vi "_CSMObj-Obtain Worker Agent.vi"(7 "Allowed Messages (Empty For All)":string[](array[string]), 8 "error in (no error)":errorcluster, 11 "Requested Name":string) -> (0 "error out":errorcluster, 3 "CSMQ Out":T1)   [LabVIEW 2017, in "Communicable State Machine.lvlib"]
uses:
  Communicable State Machine.lvlib
  _CSMObj.ctl
  _CSMObj-Info.ctl
  Typedef/_CSM_MODE.ctl
  _CSMObj-Refs.ctl
  _CSMObj-Data.ctl
  Priority Queue/Priority Queue.ctl
  Typedef/_Cross CSM State Data.ctl
  Typedef/_CSM_MSG_TYPE.ctl
  Typedef/_Cross CSM State Response.ctl
  Typedef/_CSM_Response Source Message.ctl
  Priority Queue/def-Data(LowPRI-Q).ctl
  _CSMObj-ModeData.ctl
  Typedef/_CSM Status Change Event Data.ctl
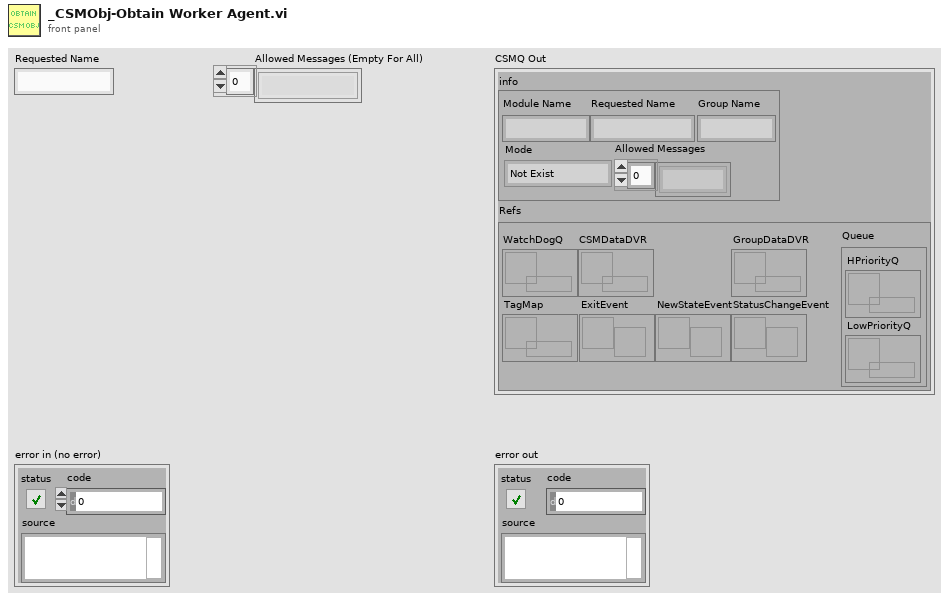
[diagram p1: front panel]
types:
  T1 = typedef "Communicable State Machine.lvlib/_CSMObj.ctl" = cluster{"info":T2, "Refs":T4}
  T2 = typedef "Communicable State Machine.lvlib/_CSMObj-Info.ctl" = cluster{"Module Name":string, "Requested Name":string, "Group Name":string, "Mode":T3, "Allowed Messages":string[]}
  T3 = typedef "Communicable State Machine.lvlib/_CSM_MODE.ctl" = enum16{"Not Exist", "Stand Alone", "CSM", "Worker", "Worker Agent", "Chain Node", "Chain"}
  T4 = typedef "Communicable State Machine.lvlib/_CSMObj-Refs.ctl" = cluster{"WatchDogQ":refnum<queue>, "CSMDataDVR":refnum<data-value>, "Queue":T5, "GroupDataDVR":refnum<data-value>, "TagMap":refnum<data-value>, "ExitEvent":refnum<user-event>, "NewStateEvent":refnum<user-event>, "StatusChangeEvent":refnum<user-event>}
  T5 = typedef "Communicable State Machine.lvlib/Priority Queue.ctl" = cluster{"HPriorityQ":refnum<queue>, "LowPriorityQ":refnum<queue>}
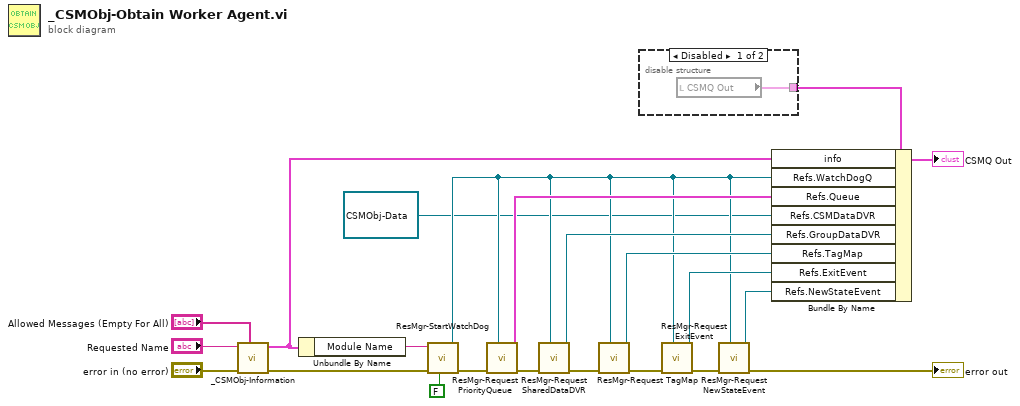
[diagram p0: block diagram]
diagram:
  n1 = call "_CSMObj-Information.vi"("Allowed Messages (Empty For All)"="Allowed Messages (Empty For All)", "Error In"="error in (no error)", "Requested Name"="Requested Name") -> ("error out"=w6:errorcluster, "CSMO-Info"=w14:T2)  [unwired: 7 in]
  n2 = Unbundle By Name(w14) -> ("Module Name"=w16:string)
  n3 = call "ResMgr-StartWatchDog.vi"("Force?"=FALSE, "error in (no error)"=w6, "ModuleName"=w16) -> ("error out"=w7:errorcluster, "WatchDogQ"=w3:refnum<queue>)  [unwired: 7 in]
  n4 = call "ResMgr-Request PriorityQueue.vi"("WatchDogQ"=w3, "Error In"=w7) -> ("error out"=w4:errorcluster, "Priority Queue"=w13:T5)  [unwired: 8 in]
  n5 = call "ResMgr-Request SharedDataDVR.vi"("WatchDogQ"=w3, "Error In"=w4) -> ("error out"=w11:errorcluster, "DVR"=w12:refnum<data-value>)  [unwired: 8 in]
  n6 = call "ResMgr-Request TagMap.vi"("WatchDogQ"=w3, "Error In"=w11) -> ("error out"=w9:errorcluster, "Data Value Reference"=w17:refnum<data-value>)  [unwired: 8 in]
  n7 = disable-structure shown="Disabled" {
    disable-tunnel: [w23 _] -> w15
    frame Disabled {
      n8 = local read "CSMQ Out"() -> (w23:T1)
    }
    frame Enabled {
    }
  }
  n9 = call "ResMgr-Request ExitEvent.vi"("WatchDogQ"=w3, "Error In"=w9) -> ("error out"=w8:errorcluster, "CSMExit"=w18:refnum<user-event>)  [unwired: 8 in]
  n10 = call "ResMgr-Request NewStateEvent.vi"("WatchDogQ"=w3, "Error In"=w8) -> ("error out"=→"error out":errorcluster, "User Event Out"=w10:refnum<user-event>)  [unwired: 8 in]
  n11 = Bundle By Name(cluster=w15, "info"=w14, "Refs.WatchDogQ"=w3, "Refs.Queue"=w13, "Refs.CSMDataDVR"=refnum<data-value> refnum ("Refs.CSM-Data"), "Refs.GroupDataDVR"=w12, "Refs.TagMap"=w17, "Refs.ExitEvent"=w18, "Refs.NewStateEvent"=w10) -> (→"CSMQ Out":T1)
